vi "Set Valve Mode.vi"(4 "time after close":u32, 6 "Valve DIR":T1, 7 "init":bool, 8 "error in (no error)":errorcluster, 11 "Stand in":refnum<class "Stand.lvclass">) -> (0 "error out":errorcluster, 2 "Done":bool)   [LabVIEW 2019, in "Stand.lvclass"]
uses:
  Stand.lvclass
  D:/GIT H4000/H4000/src/Device_class/Device.lvclass
  Valve Mode.ctl
  Device_class/Device.lvclass/Device.ctl
  FPGA/TypeDef/DO index.ctl
  Valve State Mode.vi/810e184e-eeb6-4027-a8ae-1422f3ce3d45.vi
  Valve State Mode.vi/57bd4a65-f3dc-44f5-8d68-677c2a197570.vi
  Valve State Mode.vi/03b2f9e4-fceb-4725-9b90-3fd10082a088.vi
  Valve State Mode.vi/2785bab5-dd59-4d13-b638-b9157202fa4a.vi
  Valve State Mode.vi/50faa4b8-a9b4-4cc6-ab66-55c42b424fcd.vi
  Valve State Mode.vi/c882c3fe-b7a7-4419-8f9b-6788aa23338b.vi
  Valve State Mode.vi/3d0d09bd-48e8-482f-b1e2-a36b2bb65234.vi
  Valve State Mode.vi/33d3f26a-dc4a-4f56-bf0a-61d04c5d7434.vi
  Valve State Mode.vi/52af9d47-24d1-4057-80bf-8d93bfb3d17d.vi
  Valve State Mode.vi/bbc9916c-129f-4456-975e-9c3ae3d5db66.vi
  Valve State Mode.vi/a6106d78-2bf9-477e-b655-d47fad07ddfe.vi
  Valve State Mode.vi/e2916439-03c6-4471-bb40-42242a636e27.vi
  Valve State Mode.vi/094228cb-a119-423c-9af8-5a16f059a318.vi
  Valve State Mode.vi/bf5ad1e6-a0ae-4579-ad74-ca8f304cb7cf.vi
  Valve State Mode.vi/eb4d2b76-f0f0-4e1d-bda0-609c5f37b4e7.vi
  Const All Valve.vi
  FPGA_API_class/FPGA API.lvclass
  Device_class/Device.lvclass
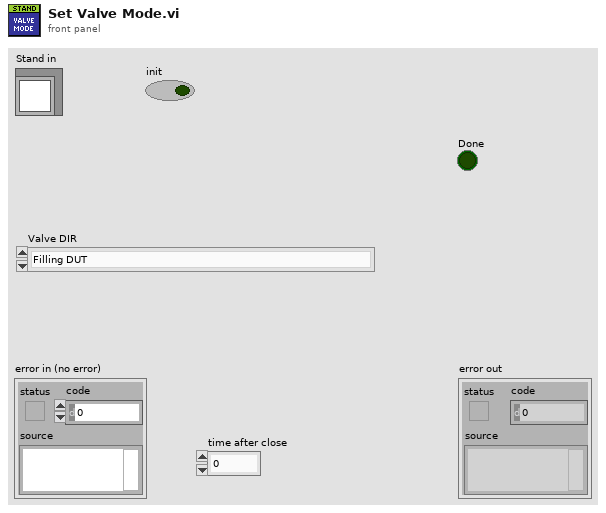
[diagram p1: front panel]
types:
  T1 = typedef "Valve Mode.ctl" = enum16{"Filling DUT", "Filling Chamber", "Pump Pressure DUT", "Pump Pressure Chamber", "Haskel Pressure DUT", "Haskel Pressure Chamber", "Slow Release DUT", "Slow Release Chamber", "Fast Release DUT", "Fast Release Chamber", "Fast Release DUT and Chamber", "Leak Pressure DUT", "Leak Pressure Chamber", "Back Pressure DUT", "Back Pressure Chamber", "Fully Closed", "Drain", "Block DUT", "Block Chamber", "filling dut down", "filling chamber down"}
  T2 = typedef "DO index.ctl" = u8
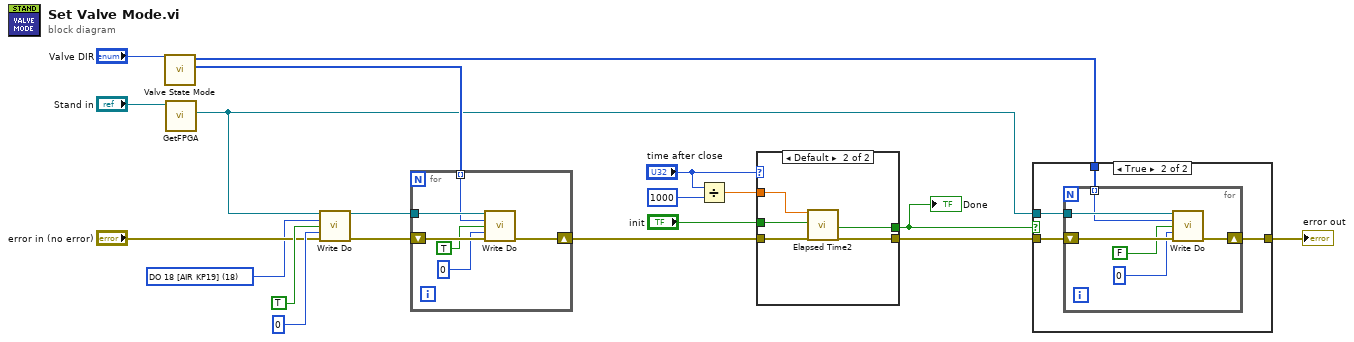
[diagram p0: block diagram]
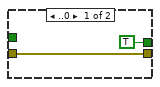
[diagram p2: hidden frame]
diagram:
  w1 = T2 18 items=["DO 0 [KP1] [M12]", "DO 1 [ON KP2] [M21]", "DO 2 [ON KP3] [M24]", "DO 3 [WATER Y18.1 [DO3]]", "DO 4 [WATER Y18.2 [DO4]]", "DO 5 [KP6 Y29.1 33.7]", "DO 6 [KP7 Y29.2 33.8]", "DO 7 [KP8 Y29.3 33.9]", "DO 8 [KP9 Y29.4  33.12]", "DO 9 [KP10 Y29.5 33.1]", "DO 10 [KP11 Y29.6 33.2]", "DO 11 [KP12 Y29.7  33.13]", "DO 12 [KP13 Y29.8  33.11]", "DO 13 [KP14 Y29.9 33.10]", "DO 14 [KP15 Y29.10  33.6]", "DO 15 [KP16 Y29.11  33.5]", "DO 16 [KP17 Y29.12  33.4]", "DO 17 [KP18 Y29.13 33.3]", "DO 18 [AIR KP19]", "DO 19 [STEP DRIVE EN KP20]", "DO 20 [KP21 Y44.1 OPEN]", "DO 21 [ KP22 Y44.1 CLOSE]", "DO 22 [ KP23 Y44.2 OPEN]", "DO 23", "DO 24 [STEP DRIVE 1]", "DO 25 [STEP DRIVE 2]"] ("#DO")
  n1 = call "Valve State Mode.vi"("Valve Mode"="Valve DIR") -> ("close"=w11:T2[], "open"=w10:T2[])  [unwired: 9 in]
  n2 = call "GetFPGA.vi"("Device in"="Stand in") -> ("FPGA API.lvclass"=w2:refnum<class "FPGA API.lvclass">)  [unwired: 10 in]
  n3 = call-dynamic "Write Do.vi"("FPGA API in"=w2, "#DO"=w1, "value"=TRUE, "Time uSec"=u32 0, "error in (no error)"="error in (no error)") -> ("FPGA API out"=w3:refnum<class "FPGA API.lvclass">, "error out"=w4:errorcluster)  [unwired: 9 in]
  n4 = for {
    shift-right: [w23] -> w19
    shift-left: w4 -> [w24]
    tunnel: w3 -> [w25]
    tunnel: w11 -> [w20] mode=indexing
    # "сначала закрыть"
    n5 = call-dynamic "Write Do.vi"("FPGA API in"=w25, "#DO"=w20, "value"=TRUE, "Time uSec"=u32 0, "error in (no error)"=w24) -> ("error out"=w23:errorcluster)  [unwired: 9 in, 1 out]
  }
  n6 = Divide(x="time after close", y=1000 ("x")) -> (x/y=w17:dbl)
  n7 = case shown="Default" "time after close" {
    tunnel: w19 -> [w27 w32]
    tunnel: [w27 w31] -> w18
    tunnel: w17 -> [_ w30]
    tunnel: [TRUE ("Time has Elapsed") w29] -> w15
    tunnel: "init" -> [_ w28]
    frame ..0 {
    }
    frame Default {
      n8 = call "Elapsed Time2"("Time Target (s)"=w30, "Reset"=w28, "error in (no error)"=w32) -> ("Time has Elapsed"=w29:bool, "error out"=w31:errorcluster)  [unwired: 9 in, 6 out]
    }
  }
  "Done" <- w15
  n9 = case shown="True" w15 {
    tunnel: [w33 w37] -> w13
    tunnel: w2 -> [_ w36]
    tunnel: w18 -> [w33 w35]
    tunnel: w10 -> [_ w34]
    frame False {
    }
    frame True {
      n10 = for {
        shift-right: [w41] -> w37
        shift-left: w35 -> [w42]
        tunnel: w36 -> [w43]
        tunnel: w34 -> [w38] mode=indexing
        n11 = call-dynamic "Write Do.vi"("FPGA API in"=w43, "#DO"=w38, "value"=FALSE, "Time uSec"=u32 0, "error in (no error)"=w42) -> ("error out"=w41:errorcluster)  [unwired: 9 in, 1 out]
      }
    }
  }
  "error out" <- w13
